vi "Teleop (1).vi"(10 "Match Info":T1={"Autonomous Elapsed Seconds"=0.0, "TeleOp Elapsed Seconds"=0.0, "Disabled Elapsed Seconds"=0.0, "Visited Autonomous"=FALSE, "Visited TeleOp"=FALSE, "Visited Disabled"=FALSE, "Autonomous Settings"={"Autonomous Style"=enum."Independent", "VI Refnum"=refnum}}, 11 "Call Context":T2) -> ()   [LabVIEW 2017]
doc: "This VI is called for each TeleOp packet received from the DS where the robot is not disabled. It is often used to read from the joysticks and update I/O or to update setpoints for timed control loops. It should complete and return within 20 milliseconds or it may miss DS packets."
uses:
  <vilib>/Rock Robotics/WPI/DriverStation/WPI_DriverStationDerivedRobotMode.ctl
  <vilib>/Rock Robotics/WPI/DriverStation/WPI_DriverStationMatch Info.ctl
  <vilib>/Rock Robotics/WPI/Solenoid/WPI_SolenoidValue.ctl
  Public/Documents/Cross The Road Electronics/Phoenix-LabVIEW/Motor Controller/Controls/CTRE_Phoenix_MotorControl_ControlMode.ctl
  <vilib>/Rock Robotics/WPI/Utilities/WPI_GetSetVariantRefNum.vi
  <vilib>/Rock Robotics/Network Tables/NT Write Boolean Array.vi
  <vilib>/Rock Robotics/Network Tables/NT Write Numeric Array.vi
  <vilib>/Rock Robotics/Network Tables/NT Read Boolean.vi
  <vilib>/Rock Robotics/Network Tables/NT Read String.vi
  <vilib>/Rock Robotics/WPI/Joystick/WPI_JoystickArcadeMapping.vi
  <vilib>/Rock Robotics/Network Tables/NT Write Number.vi
  <vilib>/Rock Robotics/WPI/RobotDrive/WPI_RobotDriveArcadeDrive_Standard(NoSaturation).vi
  <vilib>/Rock Robotics/WPI/ThirdParty/Phoenix-LabVIEW/Motor Controller/Controls/CTRE_Phoenix_MotorControl_NeutralMode.ctl
  <vilib>/Rock Robotics/Network Tables/NT Read Numeric Array.vi
  <vilib>/Rock Robotics/Network Tables/NT Read Number.vi
panel:
  out "String":string
  out "element":dbl
  in  "L Retract Ramps":bool
  in  "R Retract Ramps":bool
  in  "RRamp Raise":bool
  in  "LRamp Raise":bool=TRUE
  out "Output":bool
  in  "RRamp Deploy":bool
  in  "LRamp Deploy":bool
  in  "Cube Down":bool
  in  "Cube Up":bool
  in  "Direction Toggle":bool
  in  "Gear Shift":bool
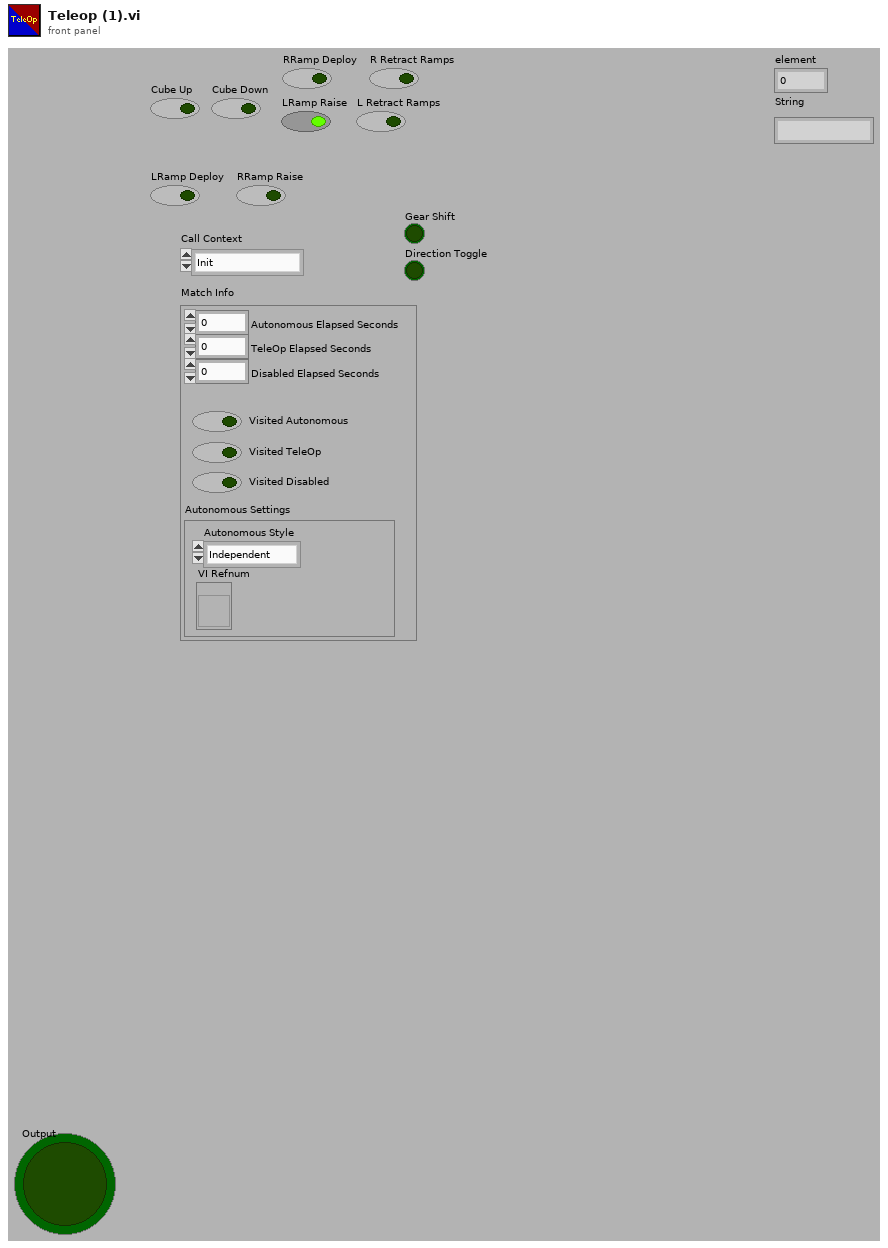
[diagram p1: front panel]
types:
  T1 = typedef "WPI_DriverStationMatch Info.ctl" = cluster{"Autonomous Elapsed Seconds":dbl, "TeleOp Elapsed Seconds":dbl, "Disabled Elapsed Seconds":dbl, "Visited Autonomous":bool, "Visited TeleOp":bool, "Visited Disabled":bool, "Autonomous Settings":cluster{"Autonomous Style":enum16{"Iterative", "Independent"}, "VI Refnum":refnum<vi>}}
  T2 = typedef "WPI_DriverStationDerivedRobotMode.ctl" = enum16{"Init", "Execute", "Stop"}
  T3 = typedef "CTRE_Phoenix_MotorControl_ControlMode.ctl" = u16
  T4 = typedef "WPI_SolenoidValue.ctl" = enum16{"Off", "On", "Forward", "Reverse"}
  T5 = typedef "WPI_JoystickDevRef.ctl" = cluster{"Device":T6}
  T6 = typedef "WPI_JoystickDeviceEnum.ctl" = enum16{"USB 0", "USB 1", "USB 2", "USB 3", "USB 4", "USB 5"}
  T7 = typedef "CTRE_Phoenix_MotorControl_NeutralMode.ctl" = enum8{"EEPROMSetting", "Override to Coast", "Override to Brake"}
  T8 = typedef "WPI_MotorControlDeviceRef.ctl" = cluster{"DeviceStatus":errorcluster, "Type":T9, "PWM":cluster{"PWM Channel":T10, "DeadBand":T11}, "CAN":cluster{"Device Number":u8, "SetOutput VI Ref":variant, "GetOutput VI Ref":variant, "Enable VI Ref":variant, "Disable VI Ref":variant, "Data":variant}, "Invert":bool, "DIO PWM":cluster{"PWM \"Enable\" Channel":T10, "DIOChannel":T12, "PWM Rate":dbl}}
  T9 = typedef "WPI_MotorControlType.ctl" = enum16{"PWM", "CAN", "DIO PWM"}
  T10 = typedef "FPGA_DIOPWMChannel.ctl" = enum8{"PWM 0", "PWM 1", "PWM 2", "PWM 3", "PWM 4", "PWM 5", "PWM 6", "PWM 7", "PWM 8", "PWM 9", "PWM MXP 0", "PWM MXP 1", "PWM MXP 2", "PWM MXP 3", "PWM MXP 4", "PWM MXP 5", "PWM MXP 6", "PWM MXP 7", "PWM MXP 8", "PWM MXP 9", "Invalid"}
  T11 = typedef "WPI_PWMDeadband.ctl" = cluster{"Name":string, "maxPositivePwm":i32, "minPositivePwm":i32, "centerPwm":i32, "maxNegativePwm":i32, "minNegativePwm":i32, "angularRange":u16}
  T12 = typedef "FPGA_DIOChannel.ctl" = enum8{"DIO 0", "DIO 1", "DIO 2", "DIO 3", "DIO 4", "DIO 5", "DIO 6", "DIO 7", "DIO 8", "DIO 9", "DIO MXP 0", "DIO MXP 1", "DIO MXP 2", "DIO MXP 3", "DIO MXP 4", "DIO MXP 5", "DIO MXP 6", "DIO MXP 7", "DIO MXP 8", "DIO MXP 9", "DIO MXP 10", "DIO MXP 11", "DIO MXP 12", "DIO MXP 13", "DIO MXP 14", "DIO MXP 15", "SPI Port CS1", "SPI Port CS2", "SPI Port CS3", "SPI Port MISO", "SPI Port MOSI", "Invalid"}
  T13 = typedef "WPI_RobotDriveDevRef.ctl" = cluster{"DevStatus":errorcluster, "Motors[]":T8[], "Square Inputs":bool, "Max Output":dbl}
  T14 = typedef "WPI_SolenoidDevRef.ctl" = cluster{"DevStatus":errorcluster, "Pneumatics Control Module":u8, "Forward Solenoid Channel":T15, "Reverse Solenoid Channel":T15}
  T15 = typedef "WPI_SolenoidChannel.ctl" = enum8{"Solenoid 0", "Solenoid 1", "Solenoid 2", "Solenoid 3", "Solenoid 4", "Solenoid 5", "Solenoid 6", "Solenoid 7", "Invalid"}
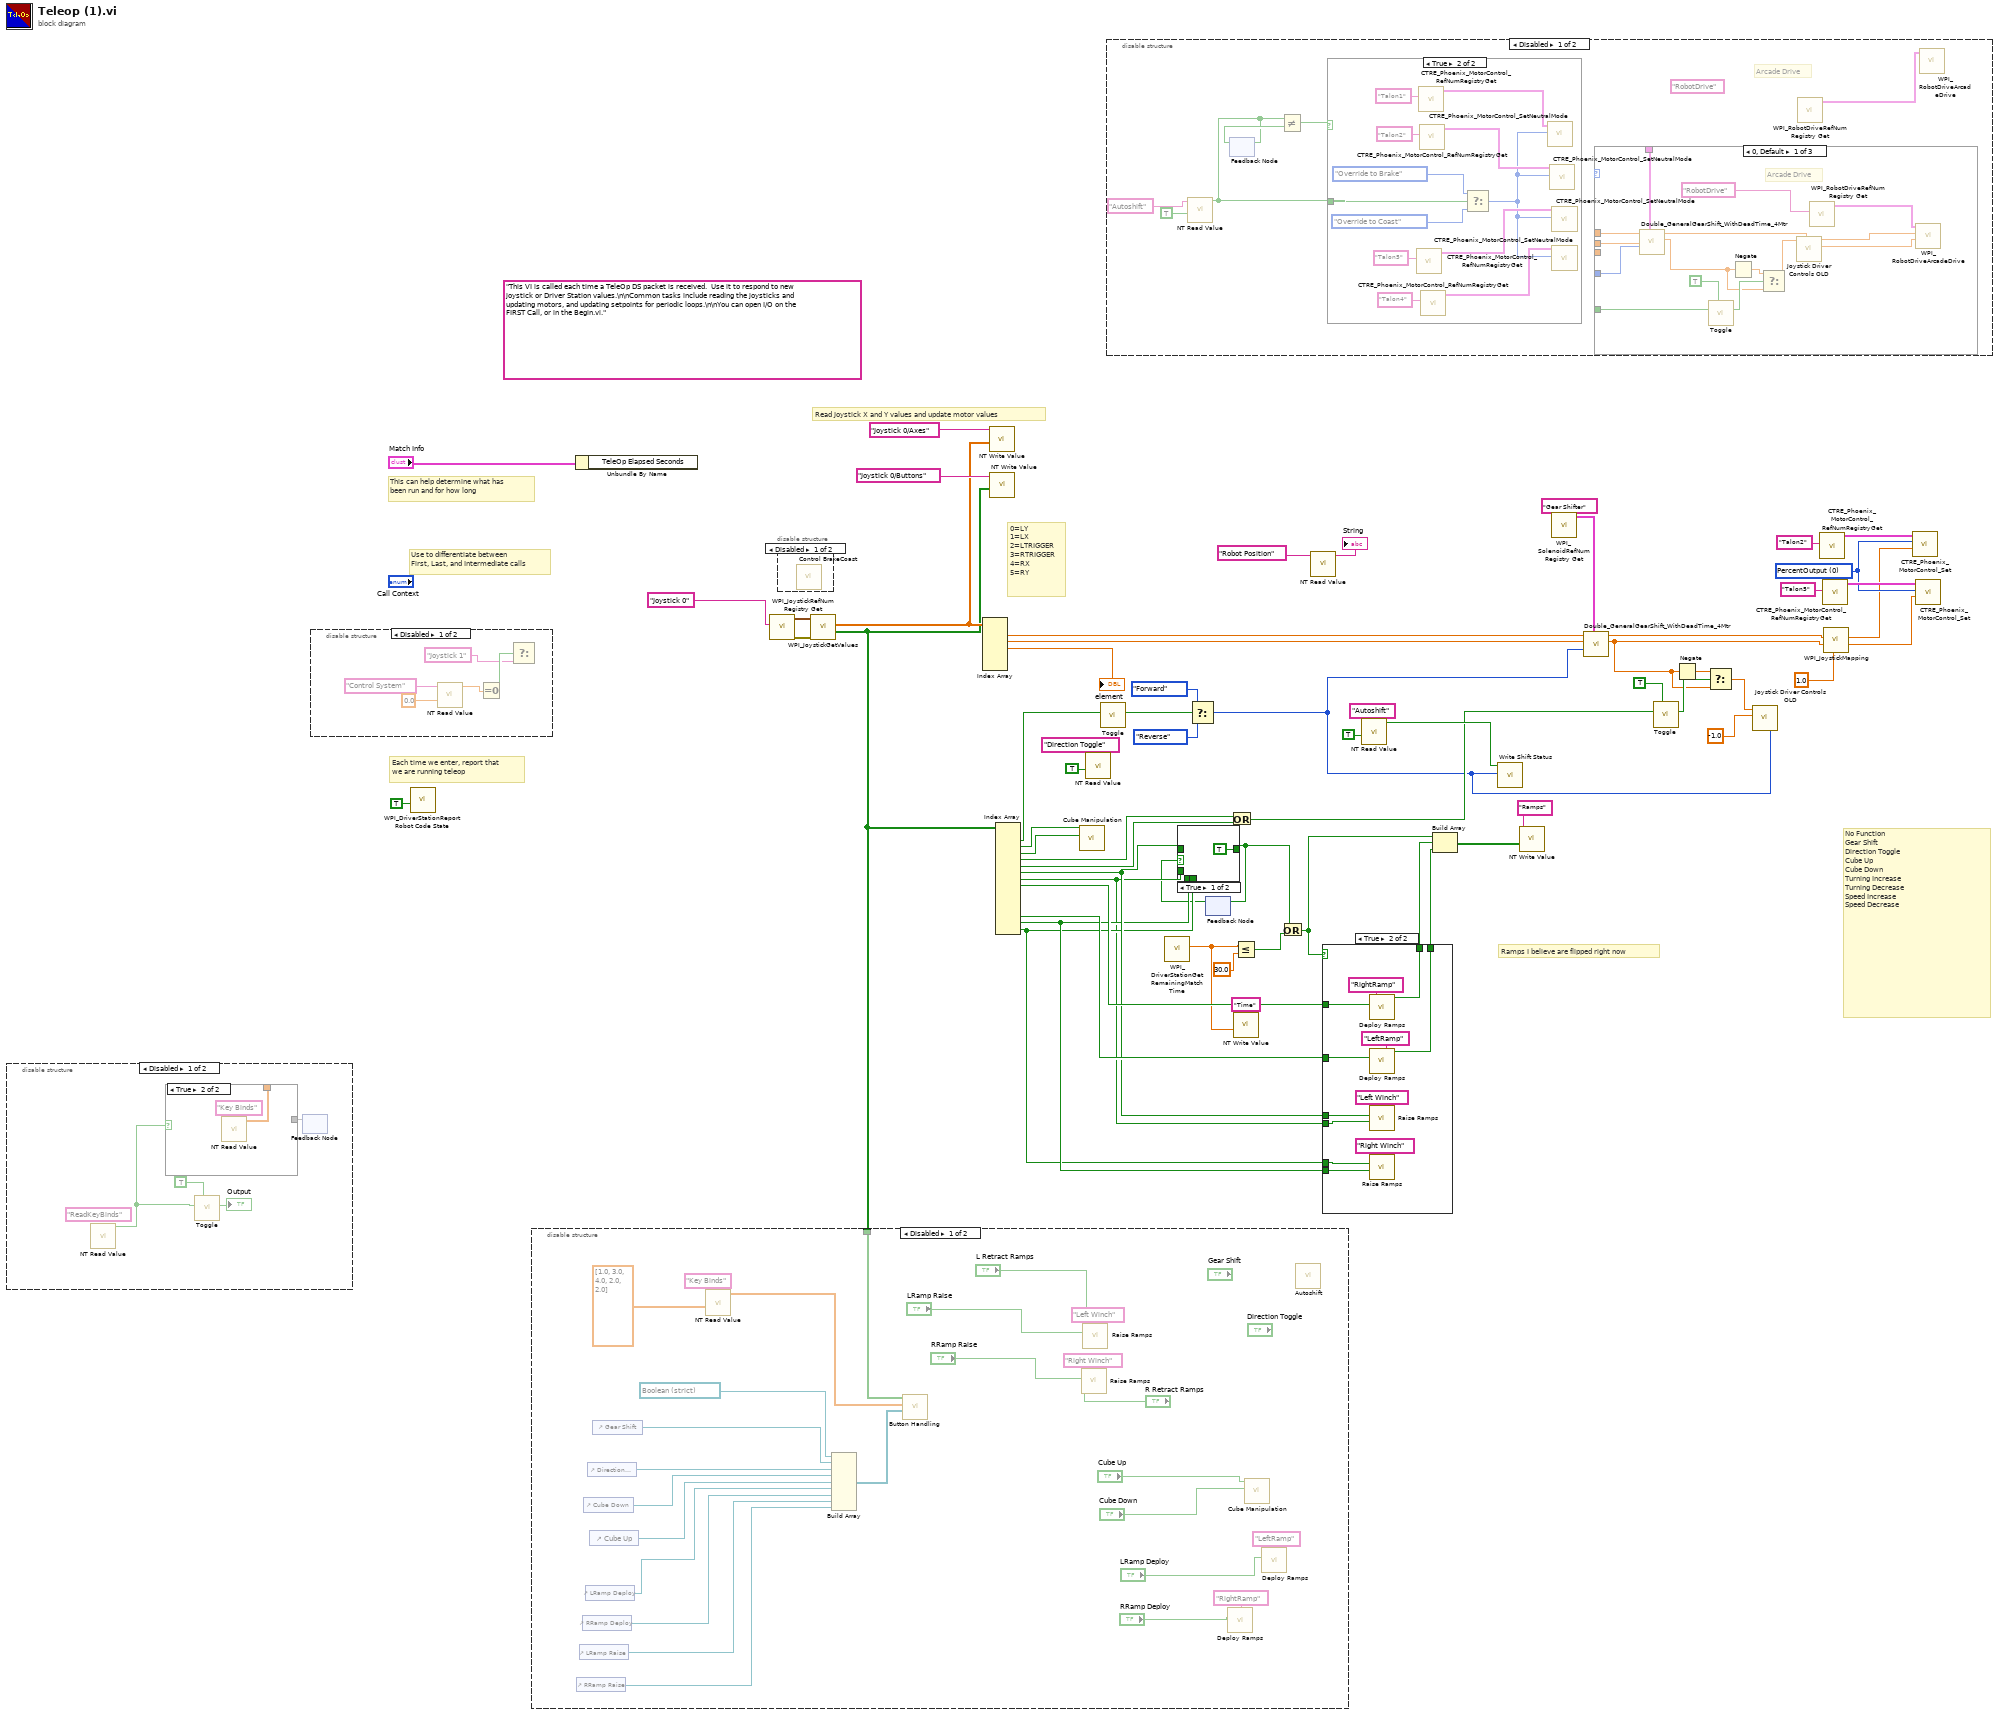
[diagram p0: block diagram]
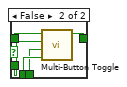
[diagram p2: hidden frame]
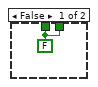
[diagram p3: hidden frame]
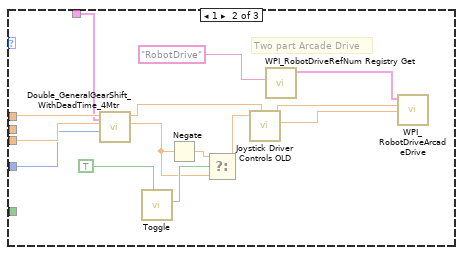
[diagram p8: hidden frame]
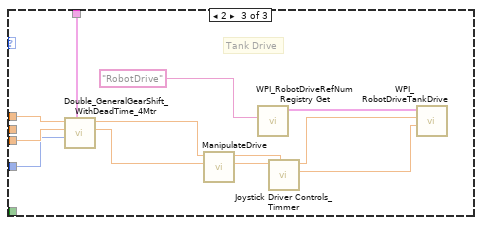
[diagram p9: hidden frame]
diagram:
  w23 = T3 0 items=["PercentOutput"=0, "Position"=1, "Velocity"=2, "Current"=3, "Follower"=5, "MotionProfile"=6, "MotionMagic"=7, "MotionMagicArc"=8, "MotionProfileArc"=10, "Disabled"=15] ("Control Mode")
  (unwired) "This VI is called each time a TeleOp DS packet is received.  Use it to respond to new joystick or Driver Station values.\n\nCommon tasks include reading the joysticks and updating motors, and updating setpoints for periodic loops.\n\nYou can open I/O on the FIRST Call, or in the Begin.vi."
  # "Ramps I believe are flipped right now"
  # "No Function\nGear Shift\nDirection Toggle\nCube Up\nCube Down\nTurning Increase\nTurning Decrease\nSpeed Increase\nSpeed Decrease"
  # "0=LY\n1=LX\n2=LTRIGGER\n3=RTRIGGER\n4=RX\n5=RY"
  # "Each time we enter, report that\nwe are running teleop"
  # "Use to differentiate between\nFirst, Last, and Intermediate calls"
  # "This can help determine what has\nbeen run and for how long"
  # "Read Joystick X and Y values and update motor values"
  n1 = disable-structure shown="Disabled" {
    frame Disabled {
      (unwired) "ReadKeyBinds" ("Name")
      n2 = call-poly <vilib>:"NT Read Value.vi"() -> ("Boolean"=w66:bool)  [unwired: 10 in, 1 out]
      n3 = call "Toggle.vi"("Control"=TRUE, "Input"=w66) -> ("Output"=→"Output":bool)  [unwired: 9 in]
      n4 = feedback #1() -> (w67)  [unwired: 1 in]
      n5 = case shown="True" w66 {
        tunnel: [w68 w69] -> _
        tunnel: w67 -> [w68 _]
        frame False {
        }
        frame True {
          n6 = call-poly <vilib>:"NT Read Value.vi"("Name"="Key Binds") -> ("Numeric Array"=w69:dbl[])  [unwired: 9 in, 1 out]
        }
      }
      n7 = feedback-in #1() -> ()  [unwired: 1 out]
    }
    frame Enabled {
    }
  }
  n8 = disable-structure shown="Disabled" {
    frame Disabled {
      n9 = call-poly <vilib>:"NT Read Value.vi"("Default Value"=0.0, "Name"="Control System") -> ("Numeric"=w73:dbl)  [unwired: 8 in, 1 out]
      n10 = Equal To 0?(x=w73) -> (x = 0?=w72:bool)
      n11 = Select(s=w72, f="Joystick 1" ("refnum name")) -> ()  [unwired: 1 in, 1 out]
    }
    frame Enabled {
    }
  }
  n12 = call <vilib>:"WPI_DriverStationReport Robot Code State.vi"("TeleOp"=TRUE ("Autonomous")) -> ()  [unwired: 10 in, 1 out]
  n13 = Unbundle By Name("Match Info") -> ()  [unwired: 1 out]
  n14 = call <vilib>:"WPI_JoystickRefNum Registry Get.vi"("refnum name"="Joystick 0") -> ("error out"=w48:errorcluster, "JoystickDevRef"=w62:T5)  [unwired: 1 in, 8 out]
  n15 = disable-structure shown="Disabled" {
    frame Disabled {
      n16 = call "Control BrakeCoast.vi"() -> ()  [unwired: 12 in]
    }
    frame Enabled {
    }
  }
  n17 = call <vilib>:"WPI_JoystickGetValues.vi"("error in (no error)"=w48, "JoystickDevRef"=w62) -> ("Buttons"=w47:bool[], "Axes"=w58:dbl[])  [unwired: 5 in, 3 out]
  n18 = disable-structure shown="Disabled" {
    disable-tunnel: w47 -> [w78 _]
    frame Disabled {
      n19 = control-ref of="RRamp Raise"() -> (w92:refnum<vi>)
      n20 = control-ref of="LRamp Raise"() -> (w93:refnum<vi>)
      n21 = control-ref of="RRamp Deploy"() -> (w95:refnum<vi>)
      n22 = control-ref of="Cube Down"() -> (w98:refnum<vi>)
      n23 = control-ref of="LRamp Deploy"() -> (w96:refnum<vi>)
      n24 = control-ref of="Direction Toggle"() -> (w100:refnum<vi>)
      n25 = control-ref of="Cube Up"() -> (w97:refnum<vi>)
      n26 = control-ref of="Gear Shift"() -> (w101:refnum<vi>)
      n27 = call-poly <vilib>:"NT Read Value.vi"("Default Value"=dbl[] [1.0, 3.0, 4.0, 2.0, 2.0], "Name"="Key Binds") -> ("Numeric Array"=w77:dbl[])  [unwired: 8 in, 1 out]
      n28 = Build Array(refnum<vi> refnum ("element"), w101, w100, w98, w97, w96, w95, w93, w92) -> (w76:refnum<vi>[])
      n29 = call "Button Handling.vi"("Array"=w76, "Numeric Array"=w77, "Buttons"=w78) -> ()  [unwired: 9 in]
      n30 = call "Raise Ramps.vi"("Retract Ramps"="R Retract Ramps", "Raise Ramps"="RRamp Raise", "refnum name"="Right Winch") -> ()  [unwired: 9 in]
      n31 = call "Raise Ramps.vi"("Retract Ramps"="L Retract Ramps", "Raise Ramps"="LRamp Raise", "refnum name"="Left Winch") -> ()  [unwired: 9 in]
      n32 = call "Deploy Ramps.vi"("Deploy"="RRamp Deploy", "refnum name"="RightRamp") -> ()  [unwired: 9 in, 1 out]
      n33 = call "Cube Manipulation.vi"("Outtake"="Cube Down", "Intake"="Cube Up") -> ()  [unwired: 10 in]
      n34 = call "Deploy Ramps.vi"("Deploy"="LRamp Deploy", "refnum name"="LeftRamp") -> ()  [unwired: 9 in, 1 out]
      n35 = call "Autoshift.vi"() -> ()  [unwired: 12 in]
    }
    frame Enabled {
    }
  }
  n36 = Index Array(array=w58) -> (element #1=w57:dbl, element #2=w56:dbl, element #3=→"element":dbl)  [unwired: 6 in, 3 out]
  n37 = call-poly <vilib>:"NT Write Value.vi"("Numeric Array"=w58, "Name"="Joystick 0/Axes") -> ()  [unwired: 9 in, 1 out]
  n38 = call-poly <vilib>:"NT Write Value.vi"("Boolean Array"=w47, "Name"="Joystick 0/Buttons") -> ()  [unwired: 9 in, 1 out]
  n39 = Index Array(array=w47) -> (element #1=w38:bool, element #2=w39:bool, element #3=w40:bool, element #4=w29:bool, element #5=w30:bool, element #6=w13:bool, element #7=w10:bool, element #8=w19:bool, element #9=w20:bool, element #10=w12:bool, element #11=w11:bool)  [unwired: 15 in, 4 out]
  n40 = call "Cube Manipulation.vi"("Outtake"=w40, "Intake"=w39) -> ()  [unwired: 10 in]
  n41 = call-poly <vilib>:"NT Read Value.vi"("Default Value"=TRUE, "Name"="Direction Toggle") -> ()  [unwired: 8 in, 2 out]
  n42 = call "Toggle.vi"("Input"=w38) -> ("Output"=w54:bool)  [unwired: 10 in]
  n43 = disable-structure shown="Disabled" {
    frame Disabled {
      (unwired) "RobotDrive" ("refnum name")
      # "Arcade Drive"
      n44 = call-poly <vilib>:"NT Read Value.vi"("Default Value"=TRUE, "Name"="Autoshift") -> ("Boolean"=w104:bool)  [unwired: 8 in, 1 out]
      n45 = feedback #2() -> (w105:bool)  [unwired: 1 in]
      n46 = feedback-in #2(w104) -> ()
      n47 = Not Equal?(x=w104, y=w105) -> (x != y?=w103:bool)
      n48 = case shown="True" w103 {
        tunnel: w104 -> [_ w156]
        frame False {
        }
        frame True {
          n49 = call <vilib>:"CTRE_Phoenix_MotorControl_RefNumRegistryGet.vi"("refnum name"="Talon5") -> ("PhoenixMotorControlDevRef"=w157:T8)  [unwired: 9 in, 1 out]
          n50 = call <vilib>:"CTRE_Phoenix_MotorControl_RefNumRegistryGet.vi"("refnum name"="Talon1") -> ("PhoenixMotorControlDevRef"=w149:T8)  [unwired: 9 in, 1 out]
          n51 = call <vilib>:"CTRE_Phoenix_MotorControl_RefNumRegistryGet.vi"("refnum name"="Talon2") -> ("PhoenixMotorControlDevRef"=w158:T8)  [unwired: 9 in, 1 out]
          n52 = call <vilib>:"CTRE_Phoenix_MotorControl_RefNumRegistryGet.vi"("refnum name"="Talon4") -> ("PhoenixMotorControlDevRef"=w151:T8)  [unwired: 9 in, 1 out]
          n53 = Select(t=CTRE_Phoenix_MotorControl_NeutralMode."Override to Brake" ("Motor Control Neutral Mode"), s=w156, f=CTRE_Phoenix_MotorControl_NeutralMode."Override to Coast" ("Motor Control Neutral Mode")) -> (s? t:f=w150:T7)
          n54 = call <vilib>:"CTRE_Phoenix_MotorControl_SetNeutralMode.vi"("Motor Control Neutral Mode"=w150, "PhoenixMotorControlDevRef"=w149) -> ()  [unwired: 8 in, 2 out]
          n55 = call <vilib>:"CTRE_Phoenix_MotorControl_SetNeutralMode.vi"("Motor Control Neutral Mode"=w150, "PhoenixMotorControlDevRef"=w158) -> ()  [unwired: 8 in, 2 out]
          n56 = call <vilib>:"CTRE_Phoenix_MotorControl_SetNeutralMode.vi"("Motor Control Neutral Mode"=w150, "PhoenixMotorControlDevRef"=w157) -> ()  [unwired: 8 in, 2 out]
          n57 = call <vilib>:"CTRE_Phoenix_MotorControl_SetNeutralMode.vi"("Motor Control Neutral Mode"=w150, "PhoenixMotorControlDevRef"=w151) -> ()  [unwired: 8 in, 2 out]
        }
      }
      n58 = case shown="0, Default" {
        selector: _ -> [_ _ _]
        tunnel: _ -> [w116 w128 w141]
        tunnel: _ -> [_ w127 w140]
        tunnel: _ -> [w115 _ _]
        tunnel: _ -> [w112 w123 w139]
        tunnel: _ -> [w111 w124 w142]
        tunnel: _ -> [w108 _ _]
        frame 0, Default {
          # "Arcade Drive"
          n59 = call "Double_GeneralGearShift_WithDeadTime_4Mtr.vi"("ShifterRef"=w111, "Shift Value"=w112, "Right"=w115, "Left"=w116) -> ("Right Output"=w113:dbl, "Left Output"=w114:dbl)  [unwired: 4 in, 2 out]
          n60 = call "Toggle.vi"("Control"=TRUE, "Input"=w108) -> ("Output"=w120:bool)  [unwired: 9 in]
          n61 = Negate(x=w113) -> (-x=w119:dbl)
          n62 = Select(t=w119, s=w120, f=w113) -> (s? t:f=w117:dbl)
          n63 = call "Joystick Driver Controls OLD.vi"("X"=w114, "Y"=w117) -> ("Y"=w110:dbl, "X"=w109:dbl)  [unwired: 8 in]
          n64 = call <vilib>:"WPI_RobotDriveRefNum Registry Get.vi"("refnum name"="RobotDrive") -> ("RobotDriveDevRef"=w121:T13)  [unwired: 9 in, 1 out]
          n65 = call-poly <vilib>:"WPI_RobotDriveArcadeDrive.vi"("Y axis value"=w110, "X axis value"=w109, "RobotDriveDevRef"=w121) -> ()  [unwired: 6 in, 3 out]
        }
        frame 1 {
          # "Two part Arcade Drive"
          n66 = call "Double_GeneralGearShift_WithDeadTime_4Mtr.vi"("ShifterRef"=w124, "Shift Value"=w123, "Right"=w127, "Left"=w128) -> ("Right Output"=w125:dbl, "Left Output"=w126:dbl)  [unwired: 4 in, 2 out]
          n67 = call "Toggle.vi"("Control"=TRUE) -> ("Output"=w132:bool)  [unwired: 10 in]
          n68 = Negate(x=w125) -> (-x=w131:dbl)
          n69 = Select(t=w131, s=w132, f=w125) -> (s? t:f=w129:dbl)
          n70 = call "Joystick Driver Controls OLD.vi"("X"=w126, "Y"=w129) -> ("Y"=w133:dbl, "X"=w134:dbl)  [unwired: 8 in]
          n71 = call <vilib>:"WPI_RobotDriveRefNum Registry Get.vi"("refnum name"="RobotDrive") -> ("RobotDriveDevRef"=w135:T13)  [unwired: 9 in, 1 out]
          n72 = call-poly <vilib>:"WPI_RobotDriveArcadeDrive.vi"("Y axis value"=w133, "X axis value"=w134, "RobotDriveDevRef"=w135) -> ()  [unwired: 6 in, 3 out]
        }
        frame 2 {
          # "Tank Drive"
          n73 = call "Double_GeneralGearShift_WithDeadTime_4Mtr.vi"("ShifterRef"=w142, "Shift Value"=w139, "Right"=w140, "Left"=w141) -> ("Right Output"=w138:dbl, "Left Output"=w137:dbl)  [unwired: 4 in, 2 out]
          n74 = call "ManipulateDrive.vi"("Y"=w138, "X"=w137) -> ("Y"=w145:dbl, "X"=w146:dbl)  [unwired: 4 in]
          n75 = call <vilib>:"WPI_RobotDriveRefNum Registry Get.vi"("refnum name"="RobotDrive") -> ("RobotDriveDevRef"=w147:T13)  [unwired: 9 in, 1 out]
          n76 = call "Joystick Driver Controls_Timmer.vi"("X"=w146, "Y"=w145) -> ("Y"=w143:dbl, "X"=w144:dbl)  [unwired: 8 in]
          n77 = call <vilib>:"WPI_RobotDriveTankDrive.vi"("Right axis value"=w143, "Left axis value"=w144, "RobotDriveDevRef"=w147) -> ()  [unwired: 6 in, 3 out]
        }
      }
      n78 = call <vilib>:"WPI_RobotDriveRefNum Registry Get.vi"() -> ("RobotDriveDevRef"=w102:T13)  [unwired: 10 in, 1 out]
      n79 = call-poly <vilib>:"WPI_RobotDriveArcadeDrive.vi"("RobotDriveDevRef"=w102) -> ()  [unwired: 8 in, 3 out]
    }
    frame Enabled {
    }
  }
  n80 = call <vilib>:"WPI_DriverStationGetRemainingMatchTime.vi"() -> ("Match Time(s)"=w9:sgl)  [unwired: 10 in, 1 out]
  n81 = Select(t=WPI_SolenoidValue."Forward" ("Shift Value"), s=w54, f=WPI_SolenoidValue."Reverse" ("Shift Value")) -> (s? t:f=w1:T4)
  n82 = feedback #3() -> (w4:bool)  [unwired: 1 in]
  n83 = case shown="True" w4 {
    tunnel: w13 -> [_ w166]
    tunnel: w12 -> [_ w165]
    tunnel: w11 -> [_ w164]
    tunnel: w10 -> [_ w163]
    tunnel: [TRUE ("Output") w162] -> w5
    frame True {
    }
    frame False {
      n84 = call "Multi-Button Toggle.vi"("Button 4"=w165, "Button 3"=w164, "Button 2"=w163, "Button 1"=w166) -> ("Output"=w162:bool)  [unwired: 7 in]
    }
  }
  n85 = feedback-in #3(w5) -> ()
  n86 = Or(x=w29, y=w30) -> (x .or. y?=w31:bool)
  n87 = Less Or Equal?(x=w9, y=sgl 30.0) -> (x <= y?=w7:bool)
  n88 = call-poly <vilib>:"NT Write Value.vi"("Numeric"=w9, "Name"="Time") -> ()  [unwired: 9 in, 1 out]
  n89 = Or(x=w5, y=w7) -> (x .or. y?=w6:bool)
  n90 = call-poly <vilib>:"NT Read Value.vi"("Name"="Robot Position") -> ("String"=→"String":string)  [unwired: 9 in, 1 out]
  n91 = case shown="True" w6 {
    tunnel: w13 -> [_ w175]
    tunnel: w10 -> [_ w174]
    tunnel: w19 -> [_ w173]
    tunnel: w20 -> [_ w172]
    tunnel: w12 -> [_ w171]
    tunnel: w11 -> [_ w170]
    tunnel: [w167 w169] -> w16
    tunnel: [w167 w168] -> w15
    frame False {
      w167 = FALSE ("Output")
    }
    frame True {
      n92 = call "Deploy Ramps.vi"("Deploy"=w173, "refnum name"="RightRamp") -> ("Output"=w169:bool)  [unwired: 9 in]
      n93 = call "Deploy Ramps.vi"("Deploy"=w172, "refnum name"="LeftRamp") -> ("Output"=w168:bool)  [unwired: 9 in]
      n94 = call "Raise Ramps.vi"("Retract Ramps"=w174, "Raise Ramps"=w175, "refnum name"="Left Winch") -> ()  [unwired: 9 in]
      n95 = call "Raise Ramps.vi"("Retract Ramps"=w171, "Raise Ramps"=w170, "refnum name"="Right Winch") -> ()  [unwired: 9 in]
    }
  }
  n96 = call-poly <vilib>:"NT Read Value.vi"("Default Value"=TRUE, "Name"="Autoshift") -> ("Boolean"=w32:bool)  [unwired: 8 in, 1 out]
  n97 = Build Array(w6, w16, w15) -> (w18:bool[])
  n98 = call "Write Shift Status.vi"("Gear"=w1, "Autoshifting"=w32) -> ()  [unwired: 9 in, 1 out]
  n99 = call-poly <vilib>:"NT Write Value.vi"("Boolean Array"=w18, "Name"="Ramps") -> ()  [unwired: 9 in, 1 out]
  n100 = call <vilib>:"WPI_SolenoidRefNum Registry Get.vi"("refnum name"="Gear Shifter") -> ("SolenoidDevRef"=w51:T14)  [unwired: 9 in, 1 out]
  n101 = call "Double_GeneralGearShift_WithDeadTime_4Mtr.vi"("ShifterRef"=w51, "Shift Value"=w1, "Right"=w56, "Left"=w57) -> ("Right Output"=w2:dbl, "Left Output"=w3:dbl)  [unwired: 4 in, 2 out]
  n102 = call "Toggle.vi"("Control"=TRUE, "Input"=w31) -> ("Output"=w46:bool)  [unwired: 9 in]
  n103 = Negate(x=w2) -> (-x=w45:dbl)
  n104 = Select(t=w45, s=w46, f=w2) -> (s? t:f=w43:dbl)
  n105 = call "Joystick Driver Controls OLD.vi"("Shift Value"=w1, "Throttle"=-1.0, "Y"=w43) -> ()  [unwired: 7 in, 2 out]
  n106 = call <vilib>:"CTRE_Phoenix_MotorControl_RefNumRegistryGet.vi"("refnum name"="Talon2") -> ("PhoenixMotorControlDevRef"=w25:T8)  [unwired: 9 in, 1 out]
  n107 = call <vilib>:"CTRE_Phoenix_MotorControl_RefNumRegistryGet.vi"("refnum name"="Talon5") -> ("PhoenixMotorControlDevRef"=w24:T8)  [unwired: 9 in, 1 out]
  n108 = call-poly <vilib>:"WPI_JoystickMapping.vi"("Max Output"=1.0, "Y axis value"=w2, "X axis value"=w3) -> ("Right Motor Value"=w22:dbl, "Left Motor Value"=w21:dbl)  [unwired: 7 in]
  n109 = call <vilib>:"CTRE_Phoenix_MotorControl_Set.vi"("Output"=w21, "Control Mode"=w23, "PhoenixMotorControlDevRef"=w25) -> ()  [unwired: 7 in, 2 out]
  n110 = call <vilib>:"CTRE_Phoenix_MotorControl_Set.vi"("Output"=w22, "Control Mode"=w23, "PhoenixMotorControlDevRef"=w24) -> ()  [unwired: 7 in, 2 out]
